vi "TIFF Get Bit Rev Table.vi"(8 "error in (no error)":errorcluster, 11 "para0":cluster{}) -> (0 "error out":errorcluster, 3 "function return":u8)   [LabVIEW 2018]
doc: "LIBTIFF_DLL_IMPEXP const unsigned char* TIFFGetBitRevTable(int);\nextern const unsigned char* TIFFGetBitRevTable(int);"
uses:
  libtiff3.dll
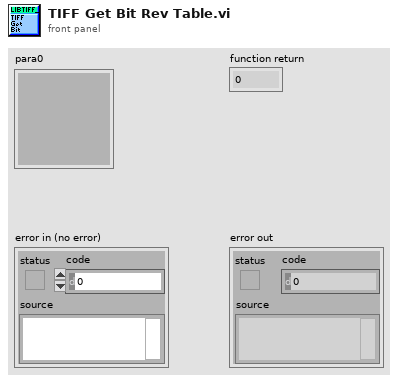
[diagram p1: front panel]
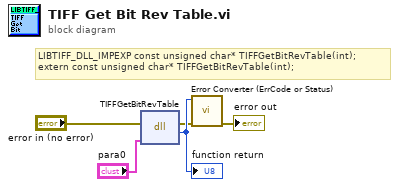
[diagram p0: block diagram]
diagram:
  # "LIBTIFF_DLL_IMPEXP\tconst unsigned char* TIFFGetBitRevTable(int);\nextern\tconst unsigned char* TIFFGetBitRevTable(int);"
  n1 = dll-call lib="C:/Users/johan/Downloads/LabVIEW software/LabVIEW software/IX-81 Software/lib/tiff/LibTiffLabview/libtiff3.*" fn="TIFFGetBitRevTable"(error in="error in (no error)", "para0"="para0") -> (error out=w2:errorcluster, w5:u8)  [unwired: 3 in, 1 out]
  "function return" <- w5
  n2 = call "Error Converter (ErrCode or Status).vi"("error in (no error)"=w2, "error code"=w5) -> ("error out"=→"error out":errorcluster)  [unwired: 9 in]
